vi "GetXMLNodeAttributes.vi"(8 "error in (no error)":errorcluster, 10 "ArributeNames":string[](array[string]), 11 "AtrributesRefIn":refnum<k20>) -> (0 "error out":errorcluster, 3 "AttributeValues":string[](array[string]))   [LabVIEW 2022 SP3]
uses:
  <vilib>/xml/Close Reference(NNMap).vi
  <vilib>/xml/Close Reference(Node).vi
  <resource>/objmgr/DOMUserDefRef.rc
  <vilib>/xml/NI_XML.lvlib
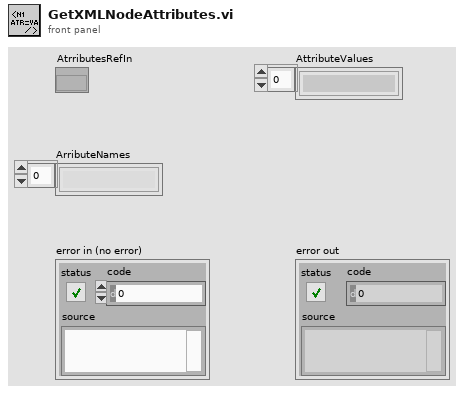
[diagram p1: front panel]
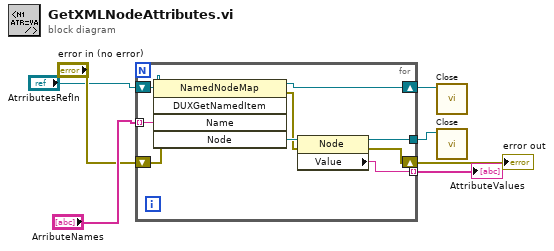
[diagram p0: block diagram]
diagram:
  n1 = for {
    tunnel: "ArributeNames" -> [w15] mode=indexing
    tunnel: [w13] -> w2 mode=indexing
    shift-right: [w10] -> w4
    shift-left: "error in (no error)" -> [w12]
    shift-right: [w9] -> w6
    shift-left: "AtrributesRefIn" -> [w16]
    tunnel: [w8] -> w7
    n2 = invoke on="Invoke Node" class="NamedNodeMap" method="DUXGetNamedItem"(reference=w16, error in=w12, "Name"=w15) -> (reference out=w9:refnum<k20>, error out=w11:errorcluster, "Node"=w14:refnum<k20>)  [unwired: 2 in, 2 out]
    n3 = property class="Node"(reference=w14, error in=w11) -> (reference out=w8:refnum<k20>, error out=w10:errorcluster, "Value"=w13:string)
  }
  "error out" <- w4
  "AttributeValues" <- w2
  n4 = call-poly <vilib>:"Close.vi"("named node map"=w6) -> ()  [unwired: 1 in, 8 out]
  n5 = call-poly <vilib>:"Close.vi"("node"=w7) -> ()  [unwired: 1 in, 8 out]
